vi "sensor buffer.vi"(6 "Channel Config":T7={"Channel Indices"=[0], "AI Max voltage"=[1.0, 1.0, 1.0, 1.0], "Calibration matrix"=[]} {"Calibration matrix"."D.O."."K" format="%.6f"; "Calibration matrix"."D.O."."Temperature" format="%.2f"; "Calibration matrix"."pH scale"."Buffers"."V/T" format="%.5f"; "Calibration matrix"."pH scale"."Buffers"."Buffer" format="%.2f"; "Calibration matrix"."pH scale"."Temperature" format="%.2f"; "Calibration matrix"."offset (physical units)" format="%.5f"; "Calibration matrix"."correspondence table"."volts" format="%.4f"; "Calibration matrix"."correspondence table"."physical units" format="%.4f"; "Calibration matrix"."second channel" min=-1; "Calibration matrix"."offset (volts)" format="%.5f"; "Calibration matrix"."conversion matrix" format="%.4e"}, 8 "command":T12, 9 "smooth interval (s)":sgl format="%.3f", 10 "max array size":u16=1 min=1, 11 "raw Data":T13 {"Sensor array" format="%.4f"; "Time" format="%<%I:%M:%S%2u %p\n%m/%d/%Y>T"}) -> (0 "Range error":bool, 1 "data rate (Hz)":sgl format="%.2f", 2 "all sensor data":T10[](array[typedef]) {"Sensor array"."scaled" format="%.2f"; "Sensor array"."voltage" format="%.4f"; "Time" format="%<%I:%M:%S%2u %p\n%m/%d/%Y>T"}, 3 "Calibrated data":T10 {"Sensor array"."scaled" format="%.2f"; "Sensor array"."voltage" format="%.4f"; "Time" format="%<%I:%M:%S%2u %p\n%m/%d/%Y>T"}, 4 "Channel Config out":T7 {"Calibration matrix"."D.O."."K" format="%.6f"; "Calibration matrix"."D.O."."Temperature" format="%.2f"; "Calibration matrix"."pH scale"."Buffers"."V/T" format="%.5f"; "Calibration matrix"."pH scale"."Buffers"."Buffer" format="%.2f"; "Calibration matrix"."pH scale"."Temperature" format="%.2f"; "Calibration matrix"."offset (physical units)" format="%.5f"; "Calibration matrix"."correspondence table"."volts" format="%.4f"; "Calibration matrix"."correspondence table"."physical units" format="%.4f"; "Calibration matrix"."second channel" min=-1; "Calibration matrix"."offset (volts)" format="%.5f"; "Calibration matrix"."conversion matrix" format="%.4e"})   [LabVIEW 2015]
doc: "Sensor buffer stores sensor data in an array. \nThe buffer must be configured using the configure command and must be given the maximum array size\n\nNew data is added to the buffer using the write command.\n\nAverage data from the last \"smooth interval\" seconds can be accessed using the average command.\n\nThe most recent data can be accessed using the recent command.\n\nThe data is arranged with the newest data at index 0."
uses:
  Distributed Daq/raw data.ctl
  TCP DAQ/Sensor data.ctl
  DAQ configuration/sensor cluster.ctl
  DAQ configuration/Sensor buffer command.ctl
  Distributed Daq/Channel config.ctl
  DAQ configuration/channel identifier.ctl
  calibration/calib array.ctl
  calibration/conversion.ctl
  DAQ configuration/scale type.ctl
  calibration/correspondence table.ctl
  calibration/pH/pH scale.ctl
  calibration/Dissolved Oxygen/DO scale.ctl
  calibration/Spectrophotometer/Photometer calibration data.ctl
panel:
  in  "Volts":T1={"conversion matrix"=[[0.0, 0.0], [0.0, 0.0], [0.0, 0.0], [0.0, 0.0], [0.0, 0.0], [0.0, 0.0]], "units"="volts", "name"="", "scale type"=enum."Volts", "offset (volts)"=0.0, "second channel"=0, "correspondence table"=[], "offset (physical units)"=0.0, "pH scale"={"Buffers"=[], "Temperature"=0.0}, "D.O."={"Temperature"=0.0, "K"=0.0, "barometric pressure"=0.0}, "Photometer data"={"Dark Voltage"=0.0, "Blank Voltage"=0.0, "Standards"=[]}} {"D.O."."K" format="%.6f"; "D.O."."Temperature" format="%.2f"; "pH scale"."Buffers"."V/T" format="%.5f"; "pH scale"."Buffers"."Buffer" format="%.2f"; "pH scale"."Temperature" format="%.2f"; "offset (physical units)" format="%.5f"; "correspondence table"."volts" format="%.4f"; "correspondence table"."physical units" format="%.4f"; "second channel" min=-1; "offset (volts)" format="%.5f"; "conversion matrix" format="%.4e"}
  # "C"
  # "kPa"
  # "C"
  # "C"
  # "kPa"
  # "C"
  # "C"
  # "kPa"
  # "C"
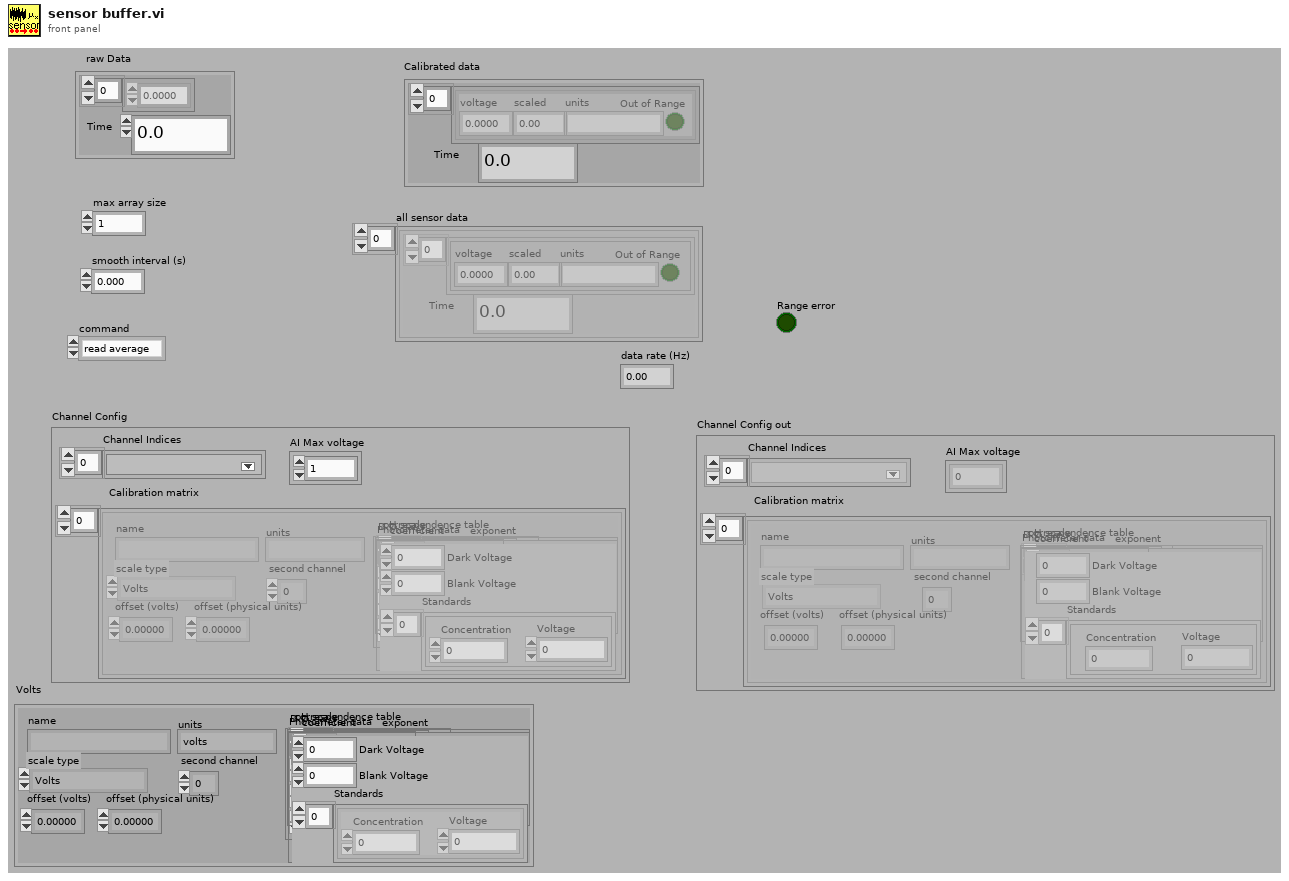
[diagram p1: front panel]
types:
  T1 = typedef "conversion.ctl" = cluster{"conversion matrix":sgl[][], "units":string, "name":string, "scale type":T2, "offset (volts)":dbl, "second channel":i8, "correspondence table":T3, "offset (physical units)":dbl, "pH scale":T4, "D.O.":T5, "Photometer data":T6}
  T2 = typedef "scale type.ctl" = enum16{"Volts", "Polynomial", "Correspondence Table", "pH", "Dissolved Oxygen", "Quadratic", "Photometer"}
  T3 = typedef "correspondence table.ctl" = cluster{"physical units":dbl, "volts":dbl}[]
  T4 = typedef "pH scale.ctl" = cluster{"Buffers":cluster{"Buffer":dbl, "Calibrated":bool, "V/T":dbl}[], "Temperature":dbl}
  T5 = typedef "DO scale.ctl" = cluster{"Temperature":dbl, "K":dbl, "barometric pressure":dbl}
  T6 = typedef "Photometer calibration data.ctl" = cluster{"Dark Voltage":dbl, "Blank Voltage":dbl, "Standards":cluster{"Concentration":dbl, "Voltage":dbl}[]}
  T7 = typedef "Channel config.ctl" = cluster{"Channel Indices":T8[], "AI Max voltage":dbl[], "Calibration matrix":T9}
  T8 = typedef "channel identifier.ctl" = u16
  T9 = typedef "calib array.ctl" = T1[]
  T10 = typedef "Sensor data.ctl" = cluster{" Sensor array":T11[], "Time":dbl}
  T11 = typedef "sensor cluster.ctl" = cluster{"voltage":sgl, "scaled":sgl, "units":string, "Out of Range":bool}
  T12 = typedef "Sensor buffer command.ctl" = enum16{"read average", "read recent", "read all", "write", "set buffer size", "Read channel config", "Write channel config", "clear"}
  T13 = typedef "raw data.ctl" = cluster{" Sensor array":sgl[], "Time":dbl}
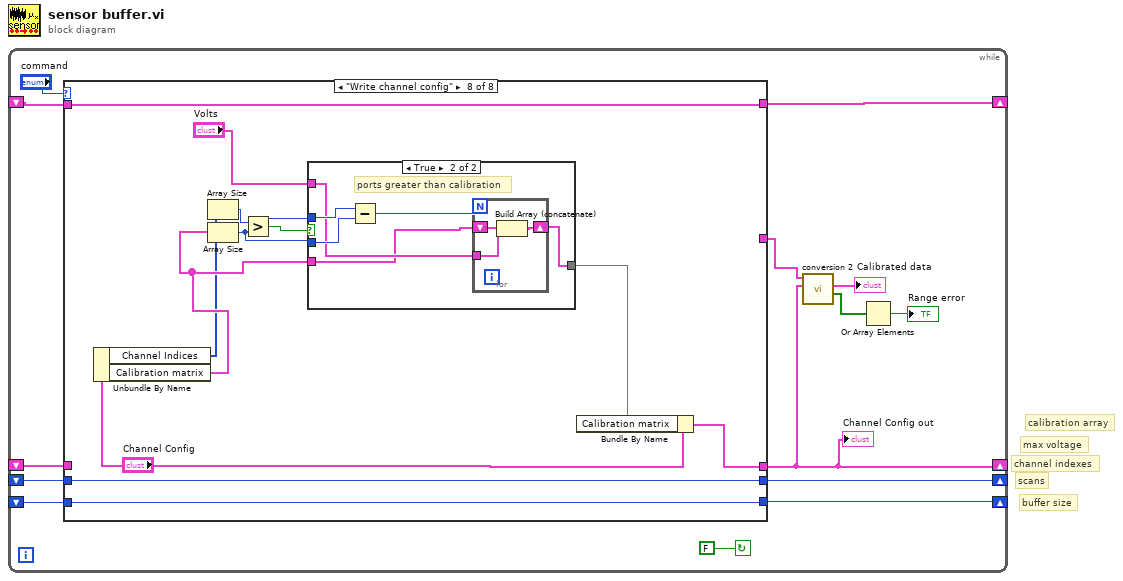
[diagram p0: block diagram]
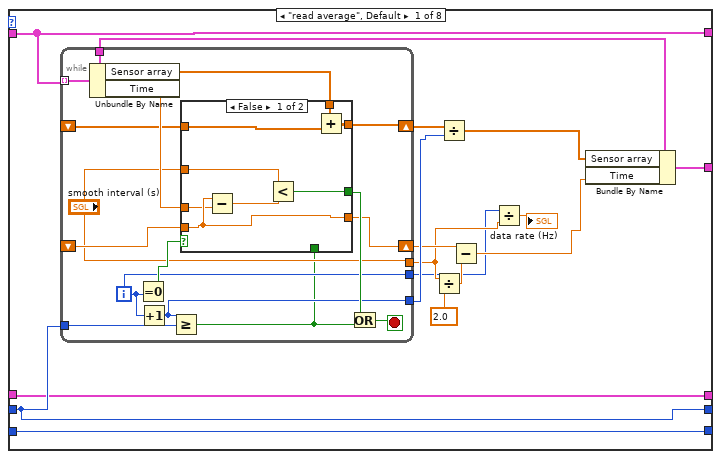
[diagram p2: hidden frame]
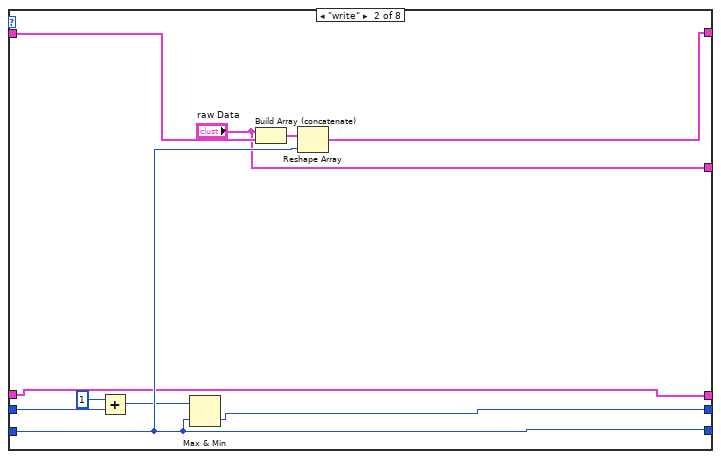
[diagram p4: hidden frame]
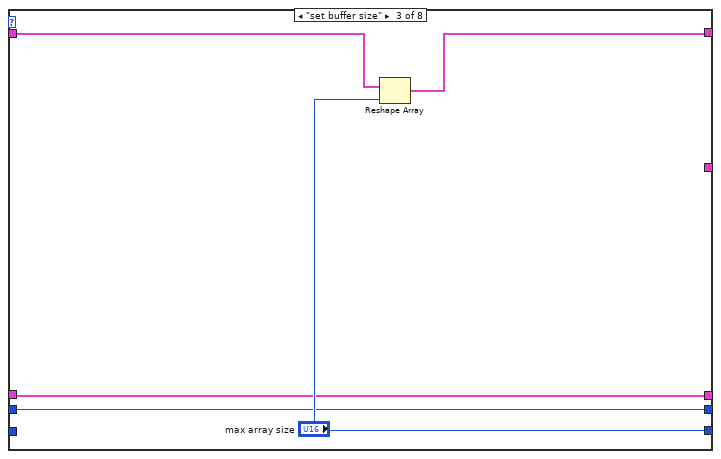
[diagram p5: hidden frame]
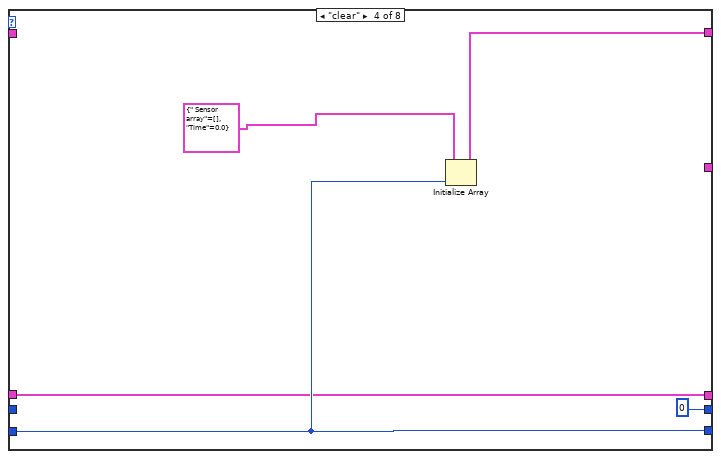
[diagram p6: hidden frame]
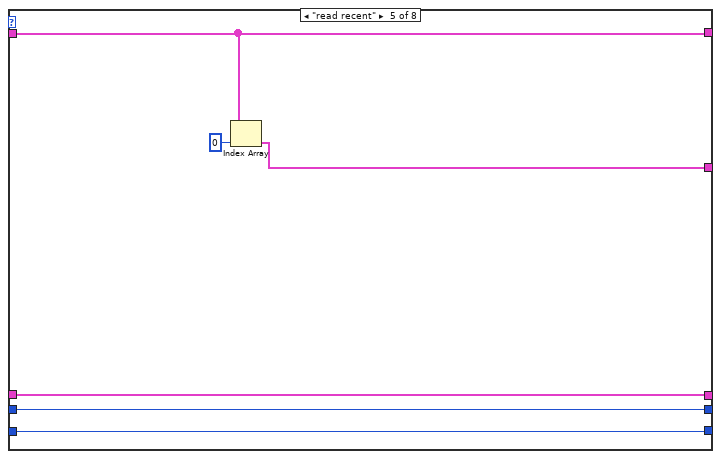
[diagram p7: hidden frame]
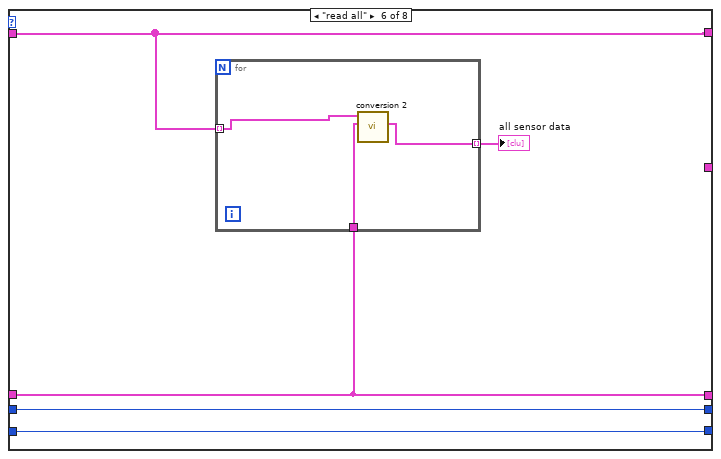
[diagram p8: hidden frame]
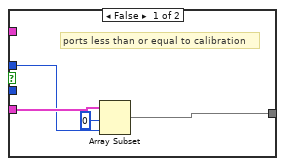
[diagram p10: hidden frame]
diagram:
  # "calibration array"
  # "max voltage"
  # "buffer size"
  # "scans"
  # "channel indexes"
  n1 = while {
    shift-right: [w13] -> _
    shift-left: _ -> [w12]
    shift-right: [w11] -> _
    shift-left: _ -> [w10]
    shift-right: [w7] -> _
    shift-left: _ -> [w8]
    shift-right: [w1] -> _
    shift-left: _ -> [w6]
    stop <- FALSE continue-if-true
    n2 = case shown="\"Write channel config\"" "command" {
      tunnel: [w21 w63 w70 w76 w82 w85 w91 w95] -> w13
      tunnel: w12 -> [w21 w65 w69 _ w82 w85 w91 w95]
      tunnel: [w30 w61 "max array size" w75 w79 w87 w94 w105] -> w11
      tunnel: w10 -> [w30 w61 _ w75 w79 w87 w94 w105]
      tunnel: [w24 "raw Data" _ _ w80 _ _ _] -> w5
      tunnel: w8 -> [w20 w64 w68 _ w78 w86 w93 w106]
      tunnel: [w20 w59 w68 0 w78 w86 w93 w106] -> w7
      tunnel: [w16 w58 w67 w72 w77 w84 w92 w96] -> w1
      tunnel: w6 -> [w16 w58 w67 w72 w77 w84 w92 _]
      frame "read average", Default {
        n3 = while {
          tunnel: w21 -> [w34] mode=indexing
          shift-right: [w33] -> w27
          shift-left: _ -> [w44]
          tunnel: w20 -> [w40]
          shift-right: [w39] -> w29
          shift-left: _ -> [w38]
          tunnel: [w35] -> w28
          tunnel: ["smooth interval (s)"] -> w19
          tunnel: [w34] -> w23
          tunnel: [w36] -> w17
          i -> [w36]
          stop <- w41 stop-if-true
          n4 = Unbundle By Name(w34) -> ("Sensor array"=w31:sgl[], "Time"=w45:dbl)
          n5 = Equal To 0?(x=w36) -> (x = 0?=w43:bool)
          n6 = Increment(x=w36) -> (x+1=w35:i32)
          n7 = Greater Or Equal?(x=w35, y=w40) -> (x >= y?=w32:bool)
          n8 = case shown="False" w43 {
            tunnel: w45 -> [w46 w56]
            tunnel: [w47 w56] -> w33
            tunnel: w44 -> [w47 _]
            tunnel: [w52 w54] -> w42
            tunnel: [w49 w55] -> w39
            tunnel: w31 -> [w51 w55]
            tunnel: w38 -> [w50 _]
            tunnel: "smooth interval (s)" -> [w48 _]
            tunnel: w32 -> [_ w54]
            frame False {
              n9 = Subtract(x=w47, y=w46) -> (x-y=w53:dbl)
              n10 = Less?(x=w48, y=w53) -> (x < y?=w52:bool)
              n11 = Add(x=w51, y=w50) -> (x+y=w49:sgl[])
            }
            frame True {
            }
          }
          n12 = Or(x=w42, y=w32) -> (x .or. y?=w41:bool)
        }
        n13 = Divide(x=w19, y=sgl 2.0) -> (x/y=w25:sgl)
        n14 = Divide(x=w29, y=w28) -> (x/y=w15:sgl[])
        n15 = Subtract(x=w27, y=w25) -> (x-y=w22:dbl)
        n16 = Divide(x=w17, y=w19) -> (x/y=→"data rate (Hz)":sgl)
        n17 = Bundle By Name(cluster=w23, "Sensor array"=w15, "Time"=w22) -> (w24:T13)
      }
      frame "write" {
        n18 = Add(x=1, y=w64) -> (x+y=w60:i32)
        n19 = Max & Min(x=w60, y=w61) -> (min(x,y)=w59:i32)  [unwired: 1 out]
        n20 = Build Array (concatenate)("raw Data", w65) -> (w62:T13[])
        n21 = Reshape Array(w62, w61) -> (w63:T13[])
      }
      frame "set buffer size" {
        n22 = Reshape Array(w69, "max array size") -> (w70:T13[])
      }
      frame "clear" {
        n23 = Initialize Array(cluster{" Sensor array":sgl[], "Time":dbl} {" Sensor array"=[], "Time"=0.0} ("raw Data"), w75) -> (w76:cluster{" Sensor array":sgl[], "Time":dbl}[])
      }
      frame "read recent" {
        n24 = Index Array(array=w82, index=0) -> (element=w80:T13)
      }
      frame "read all" {
        n25 = for {
          tunnel: w85 -> [w90] mode=indexing
          tunnel: w84 -> [w88]
          tunnel: [w89] -> w83 mode=indexing
          n26 = call "conversion 2.vi"("Channel Config"=w88, "raw Data"=w90) -> ("Calibrated data"=w89:T10)  [unwired: 7 in, 2 out]
        }
        "all sensor data" <- w83
      }
      frame "Read channel config" {
      }
      frame "Write channel config" {
        n27 = Unbundle By Name("Channel Config") -> ("Channel Indices"=w100:T8[], "Calibration matrix"=w101:T9)
        n28 = Array Size(array=w100) -> (size(s)=w104:i32)
        n29 = Array Size(array=w101) -> (size(s)=w103:i32)
        n30 = Greater?(x=w104, y=w103) -> (0:w102:bool)
        n31 = case shown="True" w102 {
          tunnel: w104 -> [w109 w116]
          tunnel: w103 -> [_ w115]
          tunnel: "Volts" -> [_ w114]
          tunnel: w101 -> [w110 w111]
          tunnel: [w107 w112] -> w98
          frame False {
            # "ports less than or equal to calibration"
            n32 = Array Subset(array=w110, index=0 ("Array Index"), length=w109) -> (w107:T9)
          }
          frame True {
            # "ports greater than calibration"
            n33 = Subtract(x=w116, y=w115) -> (x-y=w113:i32)
            n34 = for {
              N: w113 -> [_]
              tunnel: w114 -> [w119]
              shift-right: [w117] -> w112
              shift-left: w111 -> [w118]
              n35 = Build Array (concatenate)(w118, w119) -> (w117:T9)
            }
          }
        }
        n36 = Bundle By Name(cluster="Channel Config", "Calibration matrix"=w98) -> (w96:T7)
      }
    }
    "Channel Config out" <- w1
    n37 = call "conversion 2.vi"("Channel Config"=w1, "raw Data"=w5) -> ("Out of Range"=w3:bool[], "Calibrated data"=→"Calibrated data":T10)  [unwired: 7 in, 1 out]
    n38 = Or Array Elements(Boolean array=w3) -> (logical OR=→"Range error":bool)
  }
